vi "Return exe or development environment.vi"() -> (1 "exe?":bool, 2 "Application:Kind":T1(ring))   [LabVIEW 2013, in "Utility Lib.lvlib"]
doc: "This returns the application kind and a boolean which is true is the application is an exe."
uses:
  Utility Lib.lvlib
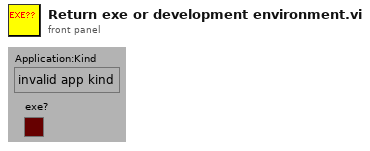
[diagram p1: front panel]
types:
  T1 = enum32{"invalid app kind", "Development System", "Run Time System", "Student Edition", "Embedded LabVIEW"}
  T2 = enum32{"invalid app kind", "Development System", "Run Time System", "Student Edition", "Embedded LabVIEW", "Evaluation", "Custom"}
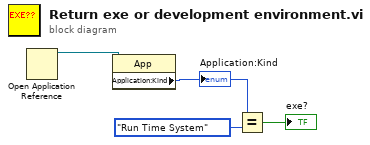
[diagram p0: block diagram]
diagram:
  n1 = Open Application Reference() -> (3:w4:refnum<vi>)  [unwired: 1 in, 4 out]
  n2 = property class="App"(reference=w4) -> ("Application:Kind"=w3:T2)  [unwired: 1 in, 2 out]
  "Application:Kind" <- w3
  n3 = Equal?(x=w3, y=T1."Run Time System") -> (x = y?=→"exe?":bool)
